vi "add_serial_ID_pair_to_part_ID_buffer.vi"(6 "recordset_in":variant[][](array[variant]), 8 "error_in":errorcluster, 10 "PART_SERIAL":string, 11 "SQL_part_ID_buffer_all_info_in":T1) -> (0 "error_out":errorcluster, 1 "PART_ID_out":string, 2 "Part exists?":bool, 3 "SQL_part_ID_buffer_all_info_out":T1)   [LabVIEW 2020]
uses:
  SQL_part_ID_buffer_all_info.ctl
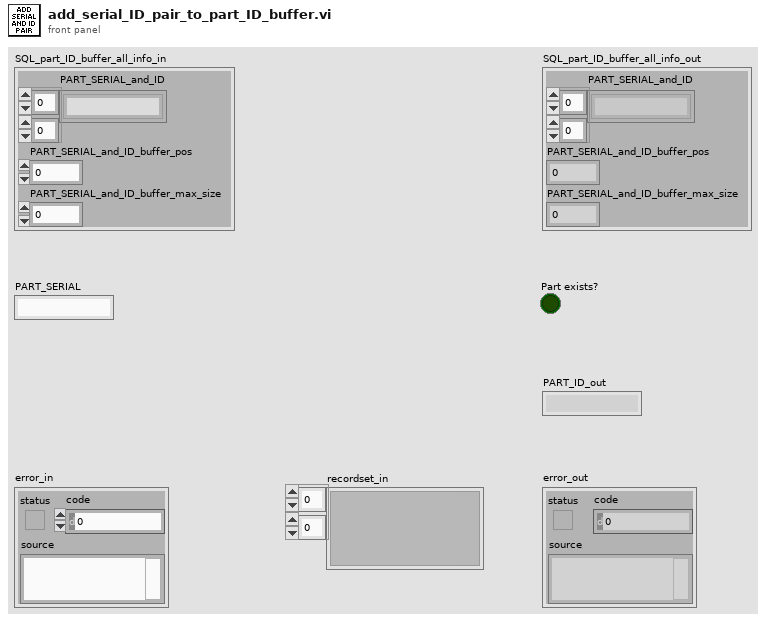
[diagram p1: front panel]
types:
  T1 = typedef "SQL_part_ID_buffer_all_info.ctl" = cluster{"PART_SERIAL_and_ID":string[][], "PART_SERIAL_and_ID_buffer_pos":i32, "PART_SERIAL_and_ID_buffer_max_size":i32}
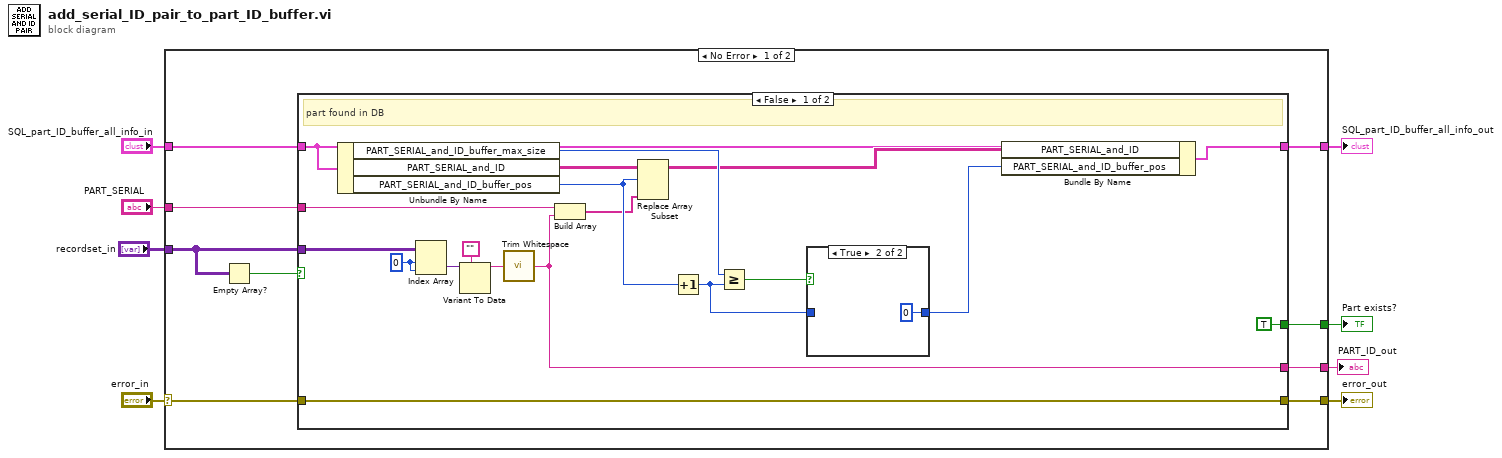
[diagram p0: block diagram]
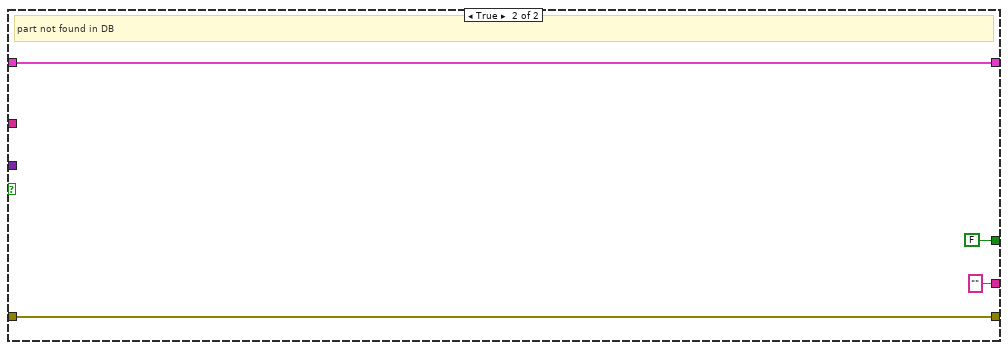
[diagram p3: hidden frame]
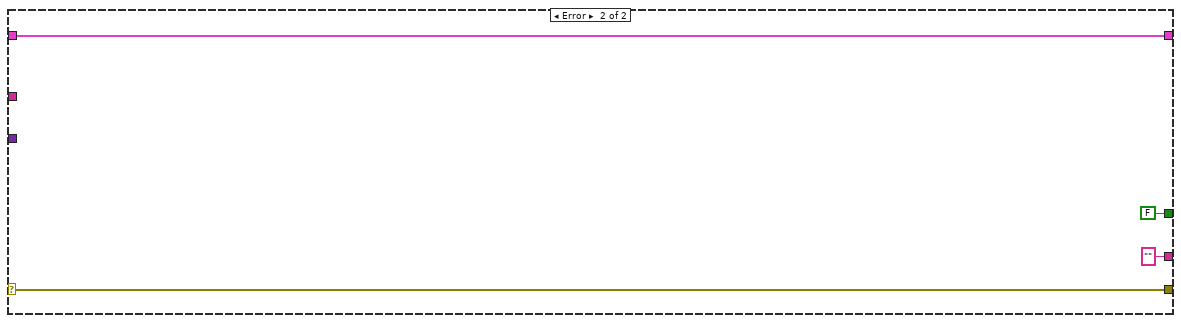
[diagram p4: hidden frame]
diagram:
  n1 = case shown="No Error" "error_in" {
    selector: "error_in" -> [w13 w46]
    tunnel: [w17 w45] -> w8
    tunnel: "SQL_part_ID_buffer_all_info_in" -> [w16 w45]
    tunnel: "PART_SERIAL" -> [w15 _]
    tunnel: [w12 w46] -> w4
    tunnel: "recordset_in" -> [w10 _]
    tunnel: [w14 "" ("trimmed string")] -> w2
    tunnel: [w11 FALSE] -> w1
    frame No Error {
      n2 = Empty Array?(array=w10) -> (empty?=w9:bool)
      n3 = case shown="False" w9 {
        tunnel: [w30 w42] -> w17
        tunnel: w16 -> [w29 w42]
        tunnel: w15 -> [w27 _]
        tunnel: w10 -> [w21 _]
        tunnel: [w20 "" ("trimmed string")] -> w14
        tunnel: w13 -> [w19 w40]
        tunnel: [w19 w40] -> w12
        tunnel: [TRUE FALSE] -> w11
        frame False {
          w22 = 0 ("index")
          # "part found in DB"
          n4 = Unbundle By Name(w29) -> ("PART_SERIAL_and_ID_buffer_max_size"=w34:i32, "PART_SERIAL_and_ID"=w26:string[][], "PART_SERIAL_and_ID_buffer_pos"=w32:i32)
          n5 = Index Array(array=w21, index (row)=w22, index (col)=w22) -> (element=w23:variant)
          n6 = Variant To Data(type="", Variant=w23) -> (data=w24:string)  [unwired: 1 in, 1 out]
          n7 = call <vilib>:"Trim Whitespace.vi"("string"=w24) -> ("trimmed string"=w20:string)  [unwired: 1 in]
          n8 = Build Array(w27, w20) -> (w28:string[])
          n9 = Replace Array Subset(array=w26, new element=w28, index (row)=w32) -> (w31:string[][])  [unwired: 1 in]
          n10 = Increment(x=w32) -> (x+1=w35:i32)
          n11 = Greater Or Equal?(x=w34, y=w35) -> (x >= y?=w33:bool)
          n12 = case shown="True" w33 {
            tunnel: w35 -> [w37 _]
            tunnel: [w37 0] -> w36
            frame False {
            }
            frame True {
            }
          }
          n13 = Bundle By Name(cluster=w29, "PART_SERIAL_and_ID"=w31, "PART_SERIAL_and_ID_buffer_pos"=w36) -> (w30:T1)
        }
        frame True {
          # "part not found in DB"
        }
      }
    }
    frame Error {
    }
  }
  "SQL_part_ID_buffer_all_info_out" <- w8
  "error_out" <- w4
  "PART_ID_out" <- w2
  "Part exists?" <- w1
